vi "Longitudinal Profile.vi"(5 "Long.X-Locations":dbl[](array[numeric])=[-500.0, -250.0, 0.0, 250.0, 500.0], 6 "Averaging time (min)":dbl, 7 "Lat.Coords":T1, 10 "Tunnel Speed":dbl, 11 "Input Task Array":T4(array[cluster])) -> (3 "Output Task Array":T4(array[cluster]))   [LabVIEW 2015]
uses:
  Anemometry Sub Vis/Gen Trav/Spacing.ctl
  Anemometry Sub Vis/Controls/Multi_run_mode.ctl
  MRCMDFBGlobal.vi
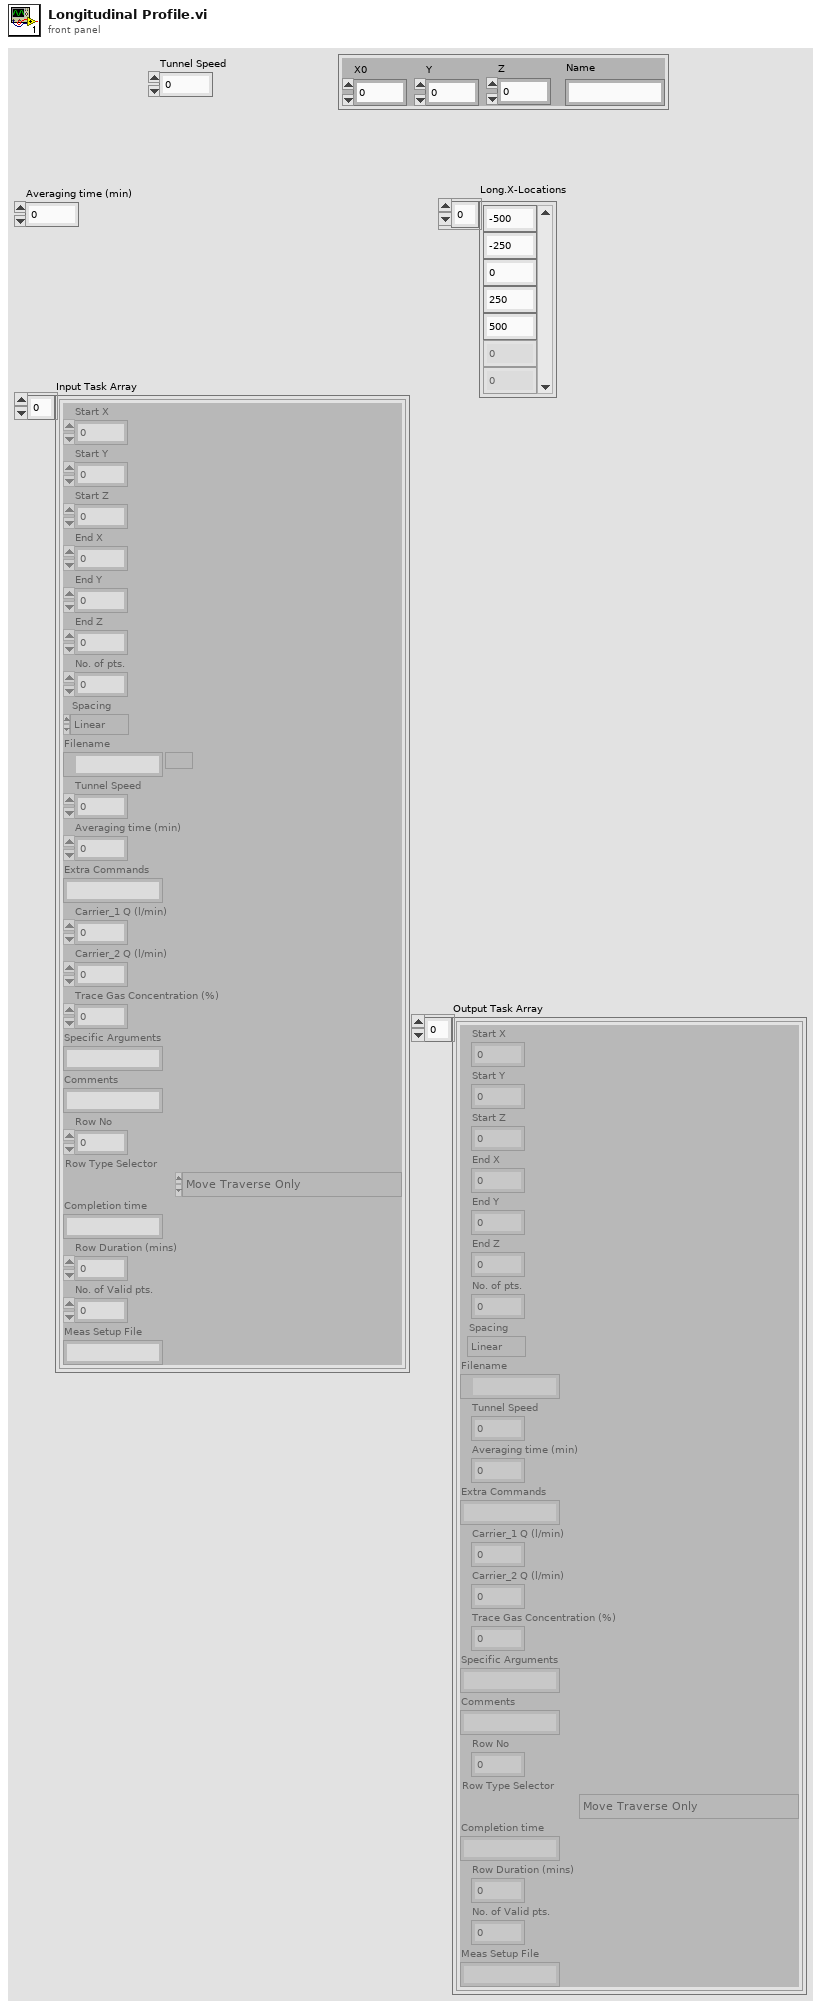
[diagram p1: front panel]
types:
  T1 = cluster{"X0":dbl, "Y":dbl, "Z":dbl, "Name":string}
  T2 = typedef "Spacing.ctl" = enum16{"Linear", "Log", "Gauss", "Specified", "N/A"}
  T3 = typedef "Multi_run_mode.ctl" = enum16{"Move Traverse Only", "Set Tunnel Speed Only", "Set Source Only", "Set Measurement Conditions", "Single Measurement", "Vertical Profile", "Lateral Profile", "Longitudinal Profile", "Explore Volume", "Multi-Axis Profile", "Auto Calibrate", "Meas Fast FID Bkgnd", "Check Beam Power", "Scanning Valve Measurement", "Run VI Named:", "Set ADAM Ch", "Wait (minutes)", "Send Message", "Synchronize With:", "Fall Back to this Row", "Turn Off Row Repeating", "Blank Row", "Traverse 3D Volume"}
  T4 = cluster{"Start X":sgl, "Start Y":sgl, "Start Z":sgl, "End X":sgl, "End Y":sgl, "End Z":sgl, "No. of pts.":i32, "Spacing":T2, "Filename":path, "Tunnel Speed":dbl, "Averaging time (min)":dbl, "Extra Commands":string, "Carrier_1 Q (l/min)":dbl, "Carrier_2 Q (l/min)":dbl, "Trace Gas Concentration (%)":dbl, "Specific Arguments":string, "Comments":string, "Row No":i32, "Row Type Selector":T3, "Completion time":string, "Row Duration (mins)":dbl, "No. of Valid pts.":i32, "Meas Setup File":string}[]
  T5 = cluster{"Start X":sgl, "Start Y":sgl, "Start Z":sgl, "End X":sgl, "End Y":sgl, "End Z":sgl, "No. of pts.":i32, "Spacing":T2, "Filename":path, "Tunnel Speed":dbl, "Averaging time (min)":dbl, "Extra Commands":string, "Carrier_1 Q (l/min)":dbl, "Carrier_2 Q (l/min)":dbl, "Trace Gas Concentration (%)":dbl, "Specific Arguments":string, "Comments":string, "Row No":i32, "Row Type Selector":T3, "Completion time":string, "Row Duration (mins)":dbl, "No. of Valid pts.":i32, "Meas Setup File":string}
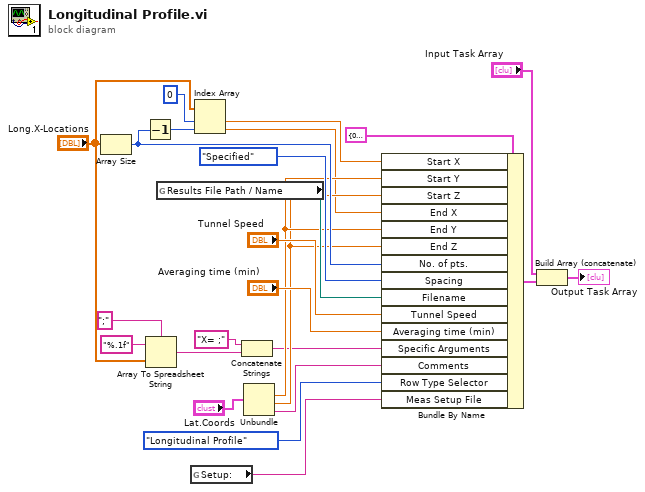
[diagram p0: block diagram]
diagram:
  n1 = Array Size(array="Long.X-Locations") -> (size(s)=w7:i32)
  n2 = Decrement(x=w7) -> (x-1=w13:i32)
  n3 = Array To Spreadsheet String(delimiter (Tab)=";", array="Long.X-Locations", 3:"%.1f" ("format string")) -> (spreadsheet string=w12:string)
  n4 = global read "MRCMDFBGlobal.vi" "Results File Path / Name"() -> (w17:path)
  n5 = global read "MRCMDFBGlobal.vi" "Setup:"() -> (w18:string)
  n6 = Index Array(array="Long.X-Locations", index #1=0 ("index"), index #2=w13) -> (element #1=w2:dbl, element #2=w3:dbl)
  n7 = Concatenate Strings("X= ;", w12) -> (w1:string)
  n8 = Unbundle("Lat.Coords") -> ("Y"=w6:dbl, "Z"=w5:dbl, "Name"=w4:string)  [unwired: 1 out]
  n9 = Bundle By Name(cluster=T5 {"Start X"=0.0, "Start Y"=0.0, "Start Z"=0.0, "End X"=0.0, "End Y"=0.0, "End Z"=0.0, "No. of pts."=0, "Spacing"=enum."Linear", "Filename"=path "", "Tunnel Speed"=0.0, "Averaging time (min)"=0.0, "Extra Commands"="", "Carrier_1 Q (l/min)"=0.0, "Carrier_2 Q (l/min)"=0.0, "Trace Gas Concentration (%)"=0.0, "Specific Arguments"="", "Comments"="", "Row No"=0, "Row Type Selector"=enum."Move Traverse Only", "Completion time"="", "Row Duration (mins)"=0.0, "No. of Valid pts."=0, "Meas Setup File"=""} ("RowTemplateConst"), "Start X"=w2, "Start Y"=w6, "Start Z"=w5, "End X"=w3, "End Y"=w6, "End Z"=w5, "No. of pts."=w7, "Spacing"=Spacing."Specified", "Filename"=w17, "Tunnel Speed"="Tunnel Speed", "Averaging time (min)"="Averaging time (min)", "Specific Arguments"=w1, "Comments"=w4, "Row Type Selector"=Multi_run_mode."Longitudinal Profile", "Meas Setup File"=w18) -> (w20:T5)
  n10 = Build Array (concatenate)("Input Task Array", w20) -> (→"Output Task Array":T4)
